vi "gluFinal.vi"() -> ()   [LabVIEW 2017]
panel:
  out "Q_old (µC)":dbl
  out "[Glu] mg/dl":dbl
  out "Vs (mV) (mV)_1":dbl
  in  "Rs (ohm)":dbl
  out "Is Glu (µA)":dbl
  out "Time  (s)":dbl
  out "Q_new (µC)":dbl
  in  "Vb (V)":dbl min=0.0 max=0.2
  out "Current in Sense Resistor":dynamicdata(graph)
  out "Vl (mV)":dbl
  out "Voltage in Load Resistor":dynamicdata(graph)
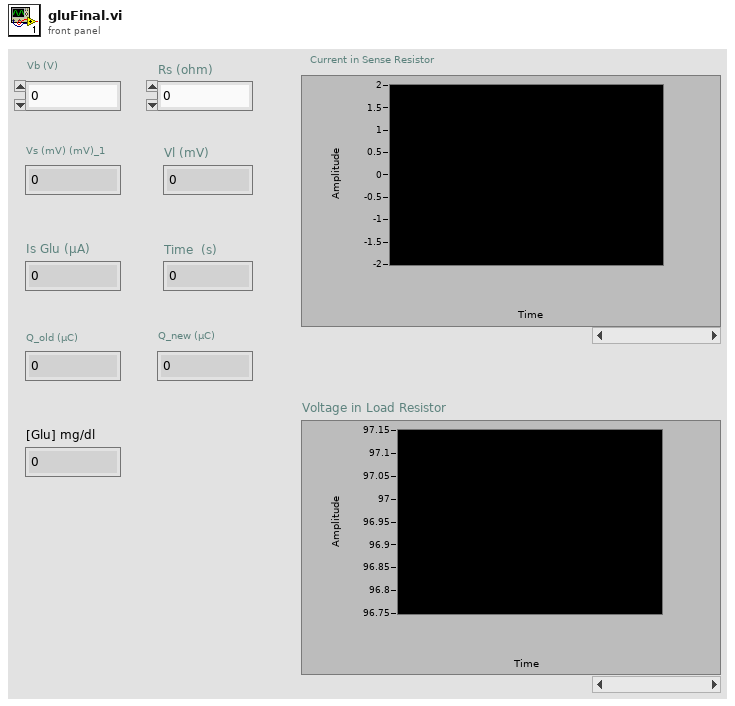
[diagram p1: front panel]
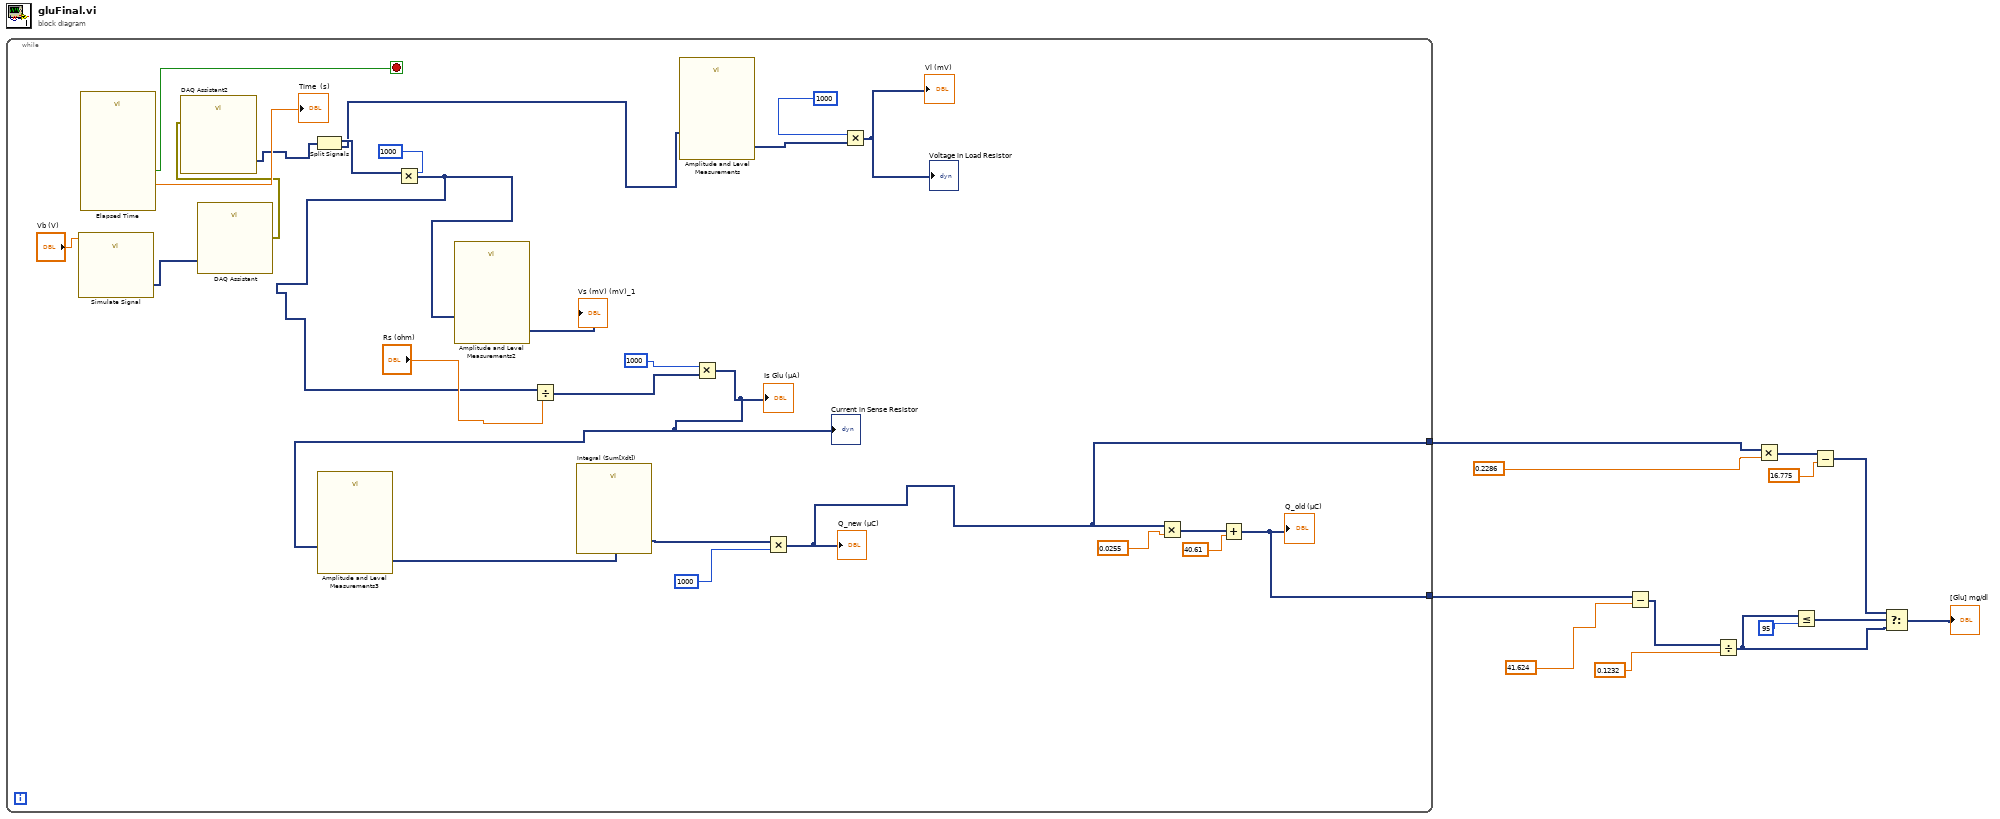
[diagram p0: block diagram]
diagram:
  n1 = while {
    tunnel: [w15] -> w2
    tunnel: [w14] -> w1
    stop <- w39 stop-if-true
    n2 = call "Simulate Signal"("Offset"="Vb (V)") -> ("DC"=w36:dynamicdata)  [unwired: 13 in, 1 out]
    n3 = call "Elapsed Time"() -> ("Elapsed Time (s)"=→"Time  (s)":dbl, "Time has Elapsed"=w39:bool)  [unwired: 12 in, 6 out]
    n4 = call "DAQ Assistant"("data"=w36) -> ("error out"=w35:errorcluster)  [unwired: 17 in, 1 out]
    n5 = call "DAQ Assistant2"("error in"=w35) -> ("data"=w30:dynamicdata)  [unwired: 16 in, 2 out]
    n6 = Split Signals(w30) -> (w29:dynamicdata, w25:dynamicdata)  [unwired: 2 in]
    n7 = Multiply(x=1000, y=w29) -> (x*y=w22:dynamicdata)
    n8 = call "Amplitude and Level Measurements2"("Signals"=w22) -> ("Mean (DC)"=→"Vs (mV) (mV)_1":dynamicdata)  [unwired: 13 in, 1 out]
    n9 = Divide(x=w22, y="Rs (ohm)") -> (x/y=w23:dynamicdata)
    n10 = call "Amplitude and Level Measurements"("Signals"=w25) -> ("Mean (DC)"=w27:dynamicdata)  [unwired: 13 in, 1 out]
    n11 = Multiply(x=1000, y=w23) -> (x*y=w19:dynamicdata)
    "Is Glu (µA)" <- w19
    "Current in Sense Resistor" <- w19
    n12 = call "Amplitude and Level Measurements3"("Signals"=w19) -> ("Mean (DC)"=w20:dynamicdata)  [unwired: 13 in, 1 out]
    n13 = call "Integral (Sum[Xdt])"("Signals"=w20) -> ("Result"=w32:dynamicdata)  [unwired: 5 in, 1 out]
    n14 = Multiply(x=w32, y=1000) -> (x*y=w14:dynamicdata)
    "Q_new (µC)" <- w14
    n15 = Multiply(x=1000, y=w27) -> (x*y=→"Vl (mV)" →"Voltage in Load Resistor":dynamicdata)
    n16 = Multiply(x=w14, y=0.0255) -> (x*y=w17:dynamicdata)
    n17 = Add(x=w17, y=40.61) -> (x+y=w15:dynamicdata)
    "Q_old (µC)" <- w15
  }
  n18 = Subtract(x=w2, y=41.624) -> (x-y=w12:dynamicdata)
  n19 = Divide(x=w12, y=0.1232) -> (x/y=w4:dynamicdata)
  n20 = Multiply(x=w1, y=0.2286) -> (x*y=w7:dynamicdata)
  n21 = Less Or Equal?(x=w4, y=95) -> (x <= y?=w6:dynamicdata)
  n22 = Subtract(x=w7, y=16.775) -> (x-y=w5:dynamicdata)
  n23 = Select(t=w5, s=w6, f=w4) -> (s? t:f=→"[Glu] mg/dl":dynamicdata)
